vi "TDMS_Rx_read.vi"(0 "Array in":u64[](array[numeric]), 5 "PDW interpoter params":T1={"Fs (Hz)"=200000000, "fft size "=4096, "F base (Hz)"=2000000000, "min AMP (dB)"=0.0, "PW low bar (fft cycle)"=0.0, "Pw high bar (fft cycle)"=7000.0, "lo likege removal (fft bin)"=-1, "max gap (fft cycle)"=0.0}) -> (4 "Array":cluster{dbl, dbl, "fixed-point":dbl, dbl}[](array[cluster]) {"?" format="%.2f"}, 8 "frequncy resolotion":dbl, 10 "PW_resolotion":dbl)   [LabVIEW 2021]
uses:
  FPGA/PDW interpoter params.ctl
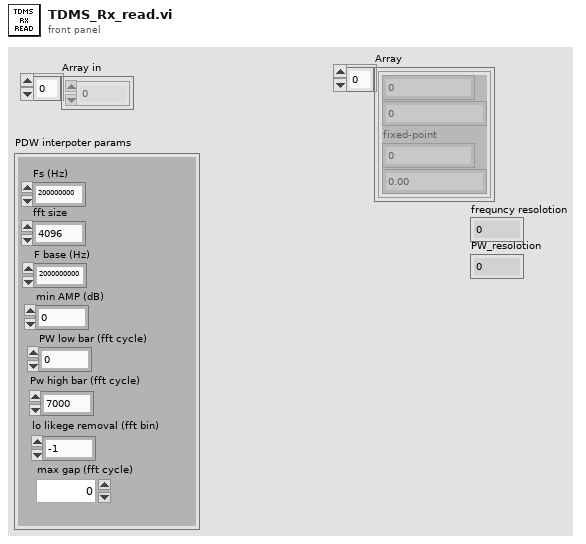
[diagram p1: front panel]
types:
  T1 = typedef "PDW interpoter params.ctl" = cluster{"Fs (Hz)":u32, "fft size ":u32, "F base (Hz)":u32, "min AMP (dB)":dbl, "PW low bar (fft cycle)":dbl, "Pw high bar (fft cycle)":dbl, "lo likege removal (fft bin)":i32, "max gap (fft cycle)":dbl}
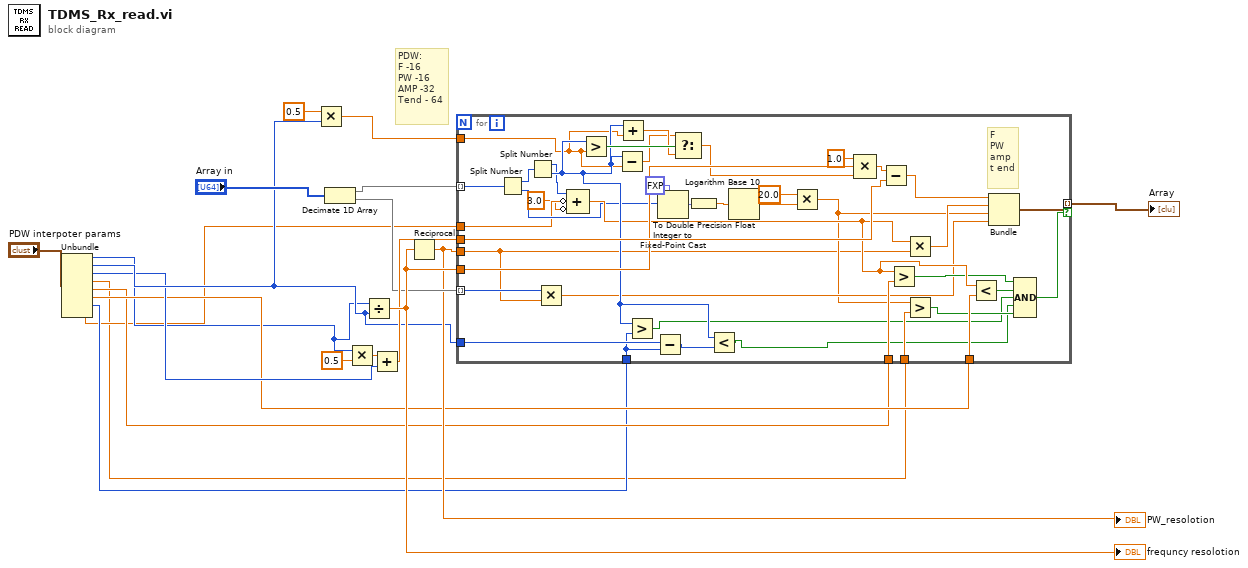
[diagram p0: block diagram]
diagram:
  # "PDW:\nF -16\nPW -16\nAMP -32\nTend - 64"
  n1 = Unbundle("PDW interpoter params") -> ("Fs (Hz)"=w5:u32, "fft size"=w8:u32, "F base (Hz)"=w7:u32, "min AMP (dB)"=w1:dbl, "PW low bar (fft cycle)"=w4:dbl, "Pw high bar (fft cycle)"=w6:dbl, "lo likege removal (fft bin)"=w3:i32, "max gap (fft cycle)"=w2:dbl)
  n2 = Multiply(x=0.5, y=w8) -> (x*y=w10:dbl)
  n3 = Decimate 1D Array("Array in") -> (w15:u64[], w14:u64[])
  n4 = Multiply(x=w5, y=0.5) -> (x*y=w18:dbl)
  n5 = Divide(x=w5, y=w8) -> (x/y=w20:dbl)
  "frequncy resolotion" <- w20
  n6 = Add(x=w18, y=w7) -> (x+y=w19:dbl)
  n7 = Reciprocal(x=w20) -> (1/x=w13:dbl)
  "PW_resolotion" <- w13
  n8 = for {
    tunnel: w15 -> [w60] mode=indexing
    tunnel: w20 -> [w57]
    tunnel: w19 -> [w58]
    tunnel: [w54] -> w12 mode=indexing if=w46
    tunnel: w13 -> [w23]
    tunnel: w4 -> [w53]
    tunnel: w6 -> [w52]
    tunnel: w14 -> [w26] mode=indexing
    tunnel: w2 -> [w37]
    tunnel: w10 -> [w36]
    tunnel: w8 -> [w34]
    tunnel: w1 -> [w27]
    tunnel: w3 -> [w22]
    # "F\nPW\namp\nt end"
    n9 = Split Number(x=w60) -> (hi(x)=w61:u32, lo(x)=w42:u32)
    n10 = Split Number(x=w61) -> (hi(x)=w44:u16, lo(x)=w45:u16)
    n11 = Multiply(x=w26, y=w23) -> (x*y=w38:dbl)
    n12 = Compound Arithmetic op=unknown(w44, invert w37, invert 3.0 ("value")) -> (w43:dbl)
    n13 = Greater?(x=w45, y=w36) -> (0:w51:bool)
    n14 = Subtract(x=w45, y=w36) -> (x-y=w49:dbl)
    n15 = Add(x=w45, y=w36) -> (x+y=w50:dbl)
    n16 = Greater?(x=w45, y=w22) -> (0:w24:bool)
    n17 = Subtract(x=w34, y=w22) -> (x-y=w35:u32)
    n18 = Integer to Fixed-Point Cast(fixed-point type=fxp<+/-,32,31> 0.0 ("fixed-point"), integer=w42) -> (fixed-point=w31:fxp<+/-,32,31>)
    n19 = Select(t=w49, s=w51, f=w50) -> (s? t:f=w48:dbl)
    n20 = To Double Precision Float(number=w31) -> (double precision float=w32:dbl)
    n21 = Less?(x=w45, y=w35) -> (x < y?=w25:bool)
    n22 = Logarithm Base 10(1:w32) -> (0:w30:dbl)
    n23 = Multiply(x=20.0, y=w30) -> (x*y=w29:dbl)
    n24 = Compound Arithmetic op=MULTIPLY(1.0 ("value"), w57, w48) -> (w59:dbl)
    n25 = Subtract(x=w59, y=w58) -> (x-y=w56:dbl)
    n26 = Greater?(x=w43, y=w53) -> (0:w40:bool)
    n27 = Multiply(x=w43, y=w23) -> (x*y=w55:dbl)
    n28 = Greater?(x=w29, y=w27) -> (0:w39:bool)
    n29 = Less?(x=w43, y=w52) -> (x < y?=w47:bool)
    n30 = Bundle(w56, w55, w29, w38) -> (w54:cluster{dbl, dbl, dbl, dbl})  [unwired: 1 in]
    n31 = Compound Arithmetic op=AND(w40, w47, w24, w25, w39) -> (w46:bool)
  }
  "Array" <- w12
